vi "GameMode.vi"(8 "error in (no error)":errorcluster, 11 "UI in":refnum<class "UI.lvclass">) -> (0 "error out":errorcluster, 3 "UI out":refnum<class "UI.lvclass">)   [LabVIEW 2019]
uses:
  User Interface/UI.lvclass
  controls/DataIn.ctl
  controls/Tabuleiro.ctl
  controls/Table.ctl
  MatchDataClasses/MatchData/MatchData.lvclass
  User Interface/UI.lvclass/UI.ctl
  User Interface/setUIData.vi
  User Interface/getUIData.vi
  User Interface/setEmbeddedVI.vi
panel:
  in  "Player 2":string
  in  "Player 1":string
  in  "Difícil":bool
  in  "Fácil":bool
  in  "Médio":bool
  in  "Multiplayer Remoto":bool
  in  "Multiplayer Local":bool
  in  "Single Player":bool
  in  "Jogar":bool
  # "Modo de Jogo"
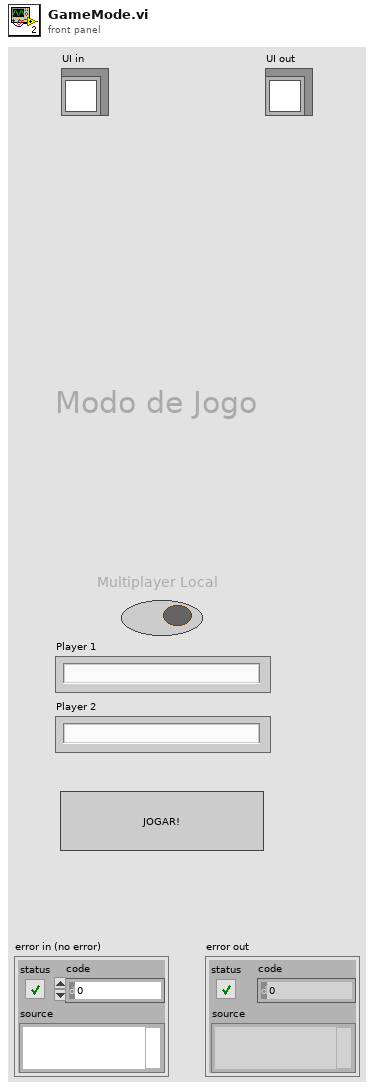
[diagram p1: front panel]
types:
  T1 = typedef "DataIn.ctl" = cluster{"Quem Joga":string, "Tabuleiro":T2, "GameOption":enum16{"Single Player", "Multiplayer local", "Multiplayer remoto", "Wait for Event", "Initialize", "Stop"}, "Turno":bool, "Player":string, "Player 1":string, "Player 2":string, "Dificuldade":enum16{"Easy", "Medium", "Hard"}, "Table":T3, "Row":u32, "Aceitar Convite":bool, "Inviter line":u32, "diretório":path, "Logout - panel close":bool, "StartGame":bool, "MatchData.lvclass":refnum<class "MatchData.lvclass">, "GameMode":enum16{"Single Easy", "Single Medium", "Single Hard", "Local", "Remote"}, "Level State":bool}
  T2 = typedef "Tabuleiro.ctl" = cluster{"(0,0)":string, "(1,0)":string, "(0,1)":string, "(1,1)":string, "(2,0)":string, "(1,2)":string, "(2,2)":string, "(0,2)":string, "(2,1) ":string}
  T3 = typedef "Table.ctl" = string[][]
  T4 = enum8{"Enabled", "Disabled", "Disabled and Grayed Out"}
  T5 = enum16{"Single Easy", "Single Medium", "Single Hard", "Local", "Remote"}
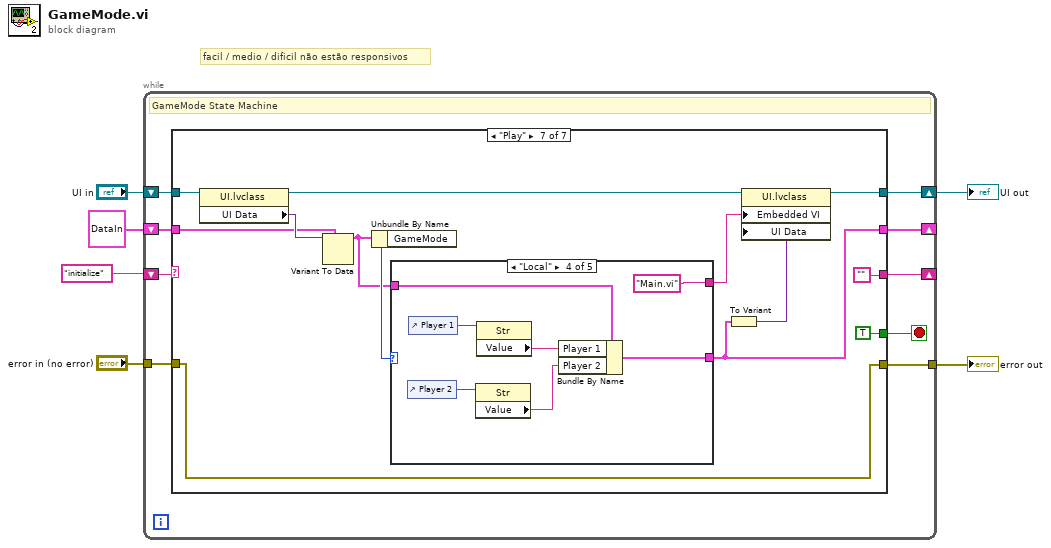
[diagram p0: block diagram]
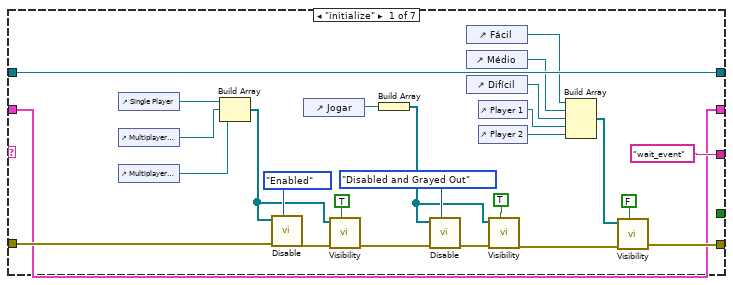
[diagram p2: hidden frame]
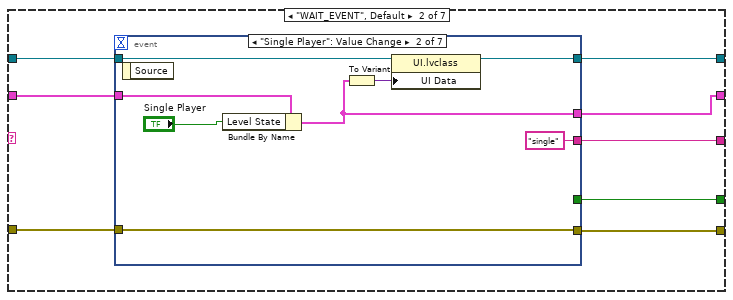
[diagram p3: hidden frame]
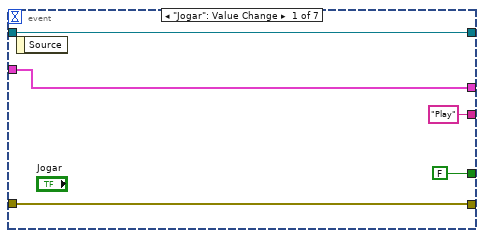
[diagram p4: hidden frame]
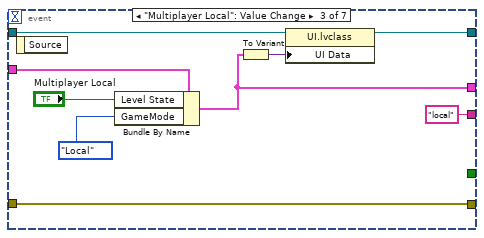
[diagram p5: hidden frame]
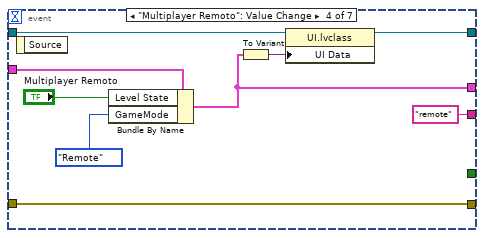
[diagram p6: hidden frame]
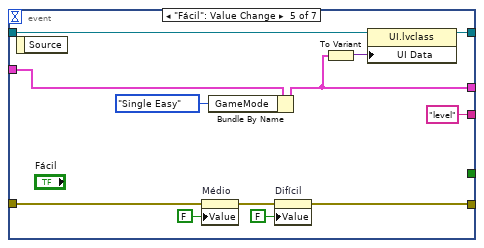
[diagram p7: hidden frame]
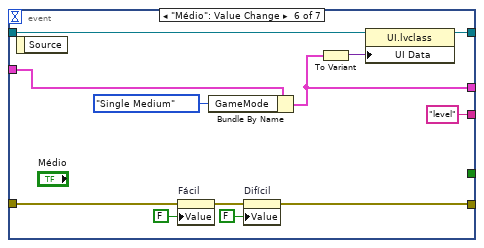
[diagram p8: hidden frame]
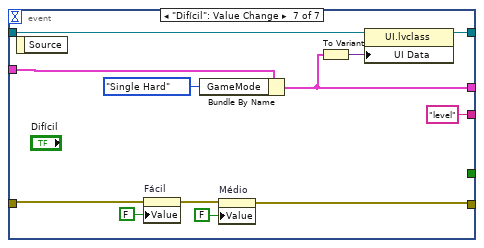
[diagram p9: hidden frame]
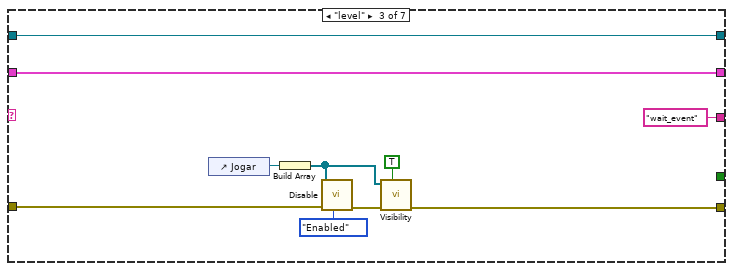
[diagram p10: hidden frame]
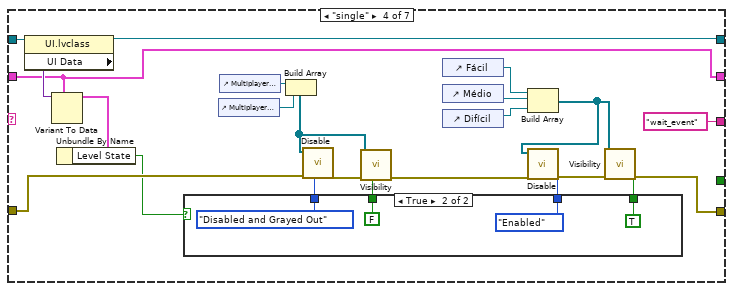
[diagram p11: hidden frame]
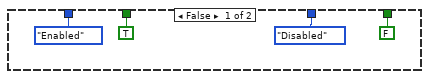
[diagram p12: hidden frame]
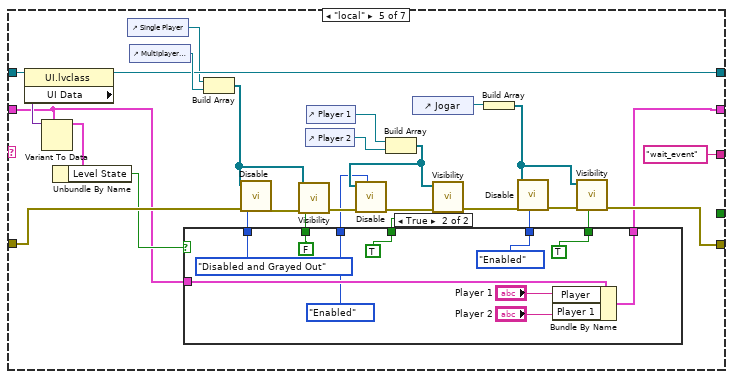
[diagram p13: hidden frame]
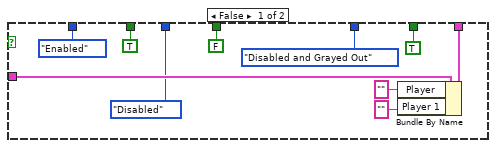
[diagram p14: hidden frame]
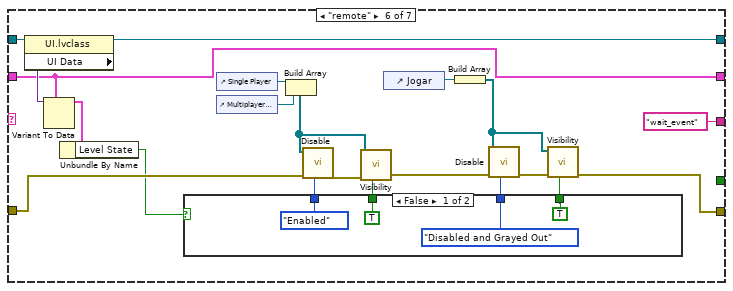
[diagram p15: hidden frame]
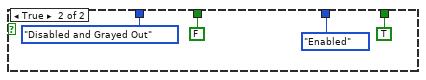
[diagram p16: hidden frame]
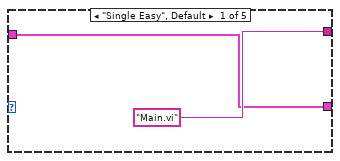
[diagram p17: hidden frame]
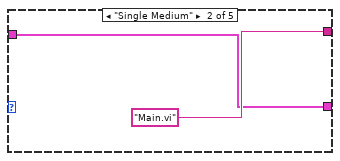
[diagram p18: hidden frame]
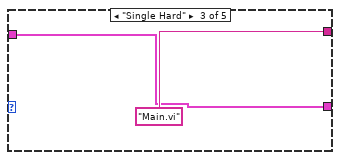
[diagram p19: hidden frame]
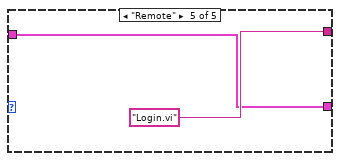
[diagram p20: hidden frame]
diagram:
  # "facil / medio / dificil não estão responsivos"
  n1 = while {
    shift-right: [w14] -> w5
    shift-left: "UI in" -> [w15]
    tunnel: [w13] -> w3
    tunnel: "error in (no error)" -> [w12]
    shift-right: [w11] -> _
    shift-left: "initialize" -> [w10]
    shift-right: [w7] -> _
    shift-left: T1 {"Quem Joga"="", "Tabuleiro"={"(0,0)"="", "(1,0)"="", "(0,1)"="", "(1,1)"="", "(2,0)"="", "(1,2)"="", "(2,2)"="", "(0,2)"="", "(2,1) "=""}, "GameOption"=enum."Multiplayer local", "Turno"=FALSE, "Player"="", "Player 1"="", "Player 2"="", "Dificuldade"=enum."Easy", "Table"=[], "Row"=0, "Aceitar Convite"=FALSE, "Inviter line"=0, "diretório"=path "", "Logout - panel close"=FALSE, "StartGame"=FALSE, "MatchData.lvclass"=refnum, "GameMode"=enum."Single Easy", "Level State"=FALSE} ("DataIn") -> [w8]
    stop <- w9 stop-if-true
    # "GameMode State Machine"
    n2 = case shown="\"Play\"" w10 {
      tunnel: w15 -> [w41 w49 w126 w133 w179 w221 w246]
      tunnel: [w41 w48 w126 w132 w178 w220 w248] -> w14
      tunnel: [w24 w47 w118 w134 w172 w213 w239] -> w13
      tunnel: w12 -> [w39 w46 w119 w142 w180 w222 w239]
      tunnel: ["wait_event" w45 "wait_event" "wait_event" "wait_event" "wait_event" ""] -> w11
      tunnel: [_ w44 _ _ _ _ TRUE] -> w9
      tunnel: w8 -> [w16 w43 w117 w130 w167 w209 w241]
      tunnel: [w16 w42 w117 w130 w166 w209 w237] -> w7
      frame "initialize" {
        n3 = control-ref of="Single Player"() -> (w37:refnum<vi>)
        n4 = control-ref of="Multiplayer Local"() -> (w36:refnum<vi>)
        n5 = control-ref of="Multiplayer Remoto"() -> (w35:refnum<vi>)
        n6 = Build Array(w37, w36, w35) -> (w33:refnum<vi>[])
        n7 = call "Disable.vi"("Disabled State"=T4."Enabled", "Error In"=w39, "Disable Controls"=w33) -> ("Error Out"=w34:errorcluster)  [unwired: 8 in]
        n8 = control-ref of="Jogar"() -> (w29:refnum<vi>)
        n9 = call "Visibility.vi"("Visible State"=TRUE, "Error In"=w34, "Visible Controls"=w33) -> ("Error Out"=w32:errorcluster)  [unwired: 8 in]
        n10 = Build Array(w29) -> (w27:refnum<vi>[])
        n11 = call "Disable.vi"("Disabled State"=T4."Disabled and Grayed Out", "Error In"=w32, "Disable Controls"=w27) -> ("Error Out"=w31:errorcluster)  [unwired: 8 in]
        n12 = control-ref of="Fácil"() -> (w18:refnum<vi>)
        n13 = control-ref of="Médio"() -> (w19:refnum<vi>)
        n14 = control-ref of="Difícil"() -> (w20:refnum<vi>)
        n15 = control-ref of="Player 1"() -> (w21:refnum<vi>)
        n16 = control-ref of="Player 2"() -> (w22:refnum<vi>)
        n17 = call "Visibility.vi"("Visible State"=TRUE, "Error In"=w31, "Visible Controls"=w27) -> ("Error Out"=w25:errorcluster)  [unwired: 8 in]
        n18 = Build Array(w18, w19, w20, w21, w22) -> (w17:refnum<vi>[])
        n19 = call "Visibility.vi"("Visible State"=FALSE, "Error In"=w25, "Visible Controls"=w17) -> ("Error Out"=w24:errorcluster)  [unwired: 8 in]
      }
      frame "WAIT_EVENT", Default {
        n20 = event shown="[1] \"Single Player\": Value Change" {
          selector: _ -> [_ _ _ _ _ _ _]
          dyn-events: _ -> [_ _ _ _ _ _ _]
          timeout: _ -> [_ _ _ _ _ _ _]
          tunnel: [w54 w59 w68 w77 w83 w96 w107] -> w48
          tunnel: w49 -> [w54 w60 w69 w78 w92 w95 w108]
          tunnel: [w53 w62 w71 w80 w88 w102 w114] -> w47
          tunnel: w46 -> [w53 w62 w71 w80 w89 w103 w116]
          tunnel: ["Play" "single" "local" "remote" "level" "level" "level"] -> w45
          tunnel: [FALSE _ _ _ _ _ _] -> w44
          tunnel: w43 -> [w50 w57 w66 w75 w85 w98 w111]
          tunnel: [w50 w55 w64 w73 w81 w93 w105] -> w42
          event "Jogar": Value Change {
            n21 = event-data() -> ()  [unwired: 1 in, 1 out]
          }
          event "Single Player": Value Change {
            n22 = event-data() -> ()  [unwired: 1 in, 1 out]
            n23 = Bundle By Name(cluster=w57, "Level State"="Single Player") -> (w55:T1)
            n24 = To Variant(anything=w55) -> (Variant=w58:variant)
            n25 = property class="UI.lvclass"(reference=w60, "UI Data"=w58) -> (reference out=w59:refnum<class "UI.lvclass">)  [unwired: 1 in, 1 out]
          }
          event "Multiplayer Local": Value Change {
            n26 = event-data() -> ()  [unwired: 1 in, 1 out]
            n27 = Bundle By Name(cluster=w66, "Level State"="Multiplayer Local", "GameMode"=T5."Local") -> (w64:T1)
            n28 = To Variant(anything=w64) -> (Variant=w67:variant)
            n29 = property class="UI.lvclass"(reference=w69, "UI Data"=w67) -> (reference out=w68:refnum<class "UI.lvclass">)  [unwired: 1 in, 1 out]
          }
          event "Multiplayer Remoto": Value Change {
            n30 = event-data() -> ()  [unwired: 1 in, 1 out]
            n31 = Bundle By Name(cluster=w75, "Level State"="Multiplayer Remoto", "GameMode"=T5."Remote") -> (w73:T1)
            n32 = To Variant(anything=w73) -> (Variant=w76:variant)
            n33 = property class="UI.lvclass"(reference=w78, "UI Data"=w76) -> (reference out=w77:refnum<class "UI.lvclass">)  [unwired: 1 in, 1 out]
          }
          event "Fácil": Value Change {
            n34 = event-data() -> ()  [unwired: 1 in, 1 out]
            n35 = property on="Médio" class="Bool (strict)"(error in=w89, "Value"=FALSE ("Médio")) -> (error out=w90:errorcluster)  [unwired: 1 in, 1 out]
            n36 = Bundle By Name(cluster=w85, "GameMode"=T5."Single Easy") -> (w81:T1)
            n37 = property on="Difícil" class="Bool (strict)"(error in=w90, "Value"=FALSE ("Difícil")) -> (error out=w88:errorcluster)  [unwired: 1 in, 1 out]
            n38 = To Variant(anything=w81) -> (Variant=w82:variant)
            n39 = property class="UI.lvclass"(reference=w92, "UI Data"=w82) -> (reference out=w83:refnum<class "UI.lvclass">)  [unwired: 1 in, 1 out]
          }
          event "Médio": Value Change {
            n40 = event-data() -> ()  [unwired: 1 in, 1 out]
            n41 = property on="Fácil" class="Bool (strict)"(error in=w103, "Value"=FALSE ("Fácil")) -> (error out=w104:errorcluster)  [unwired: 1 in, 1 out]
            n42 = Bundle By Name(cluster=w98, "GameMode"=T5."Single Medium") -> (w93:T1)
            n43 = property on="Difícil" class="Bool (strict)"(error in=w104, "Value"=FALSE ("Difícil")) -> (error out=w102:errorcluster)  [unwired: 1 in, 1 out]
            n44 = To Variant(anything=w93) -> (Variant=w94:variant)
            n45 = property class="UI.lvclass"(reference=w95, "UI Data"=w94) -> (reference out=w96:refnum<class "UI.lvclass">)  [unwired: 1 in, 1 out]
          }
          event "Difícil": Value Change {
            n46 = event-data() -> ()  [unwired: 1 in, 1 out]
            n47 = property on="Fácil" class="Bool (strict)"(error in=w116, "Value"=FALSE ("Fácil")) -> (error out=w115:errorcluster)  [unwired: 1 in, 1 out]
            n48 = Bundle By Name(cluster=w111, "GameMode"=T5."Single Hard") -> (w105:T1)
            n49 = property on="Médio" class="Bool (strict)"(error in=w115, "Value"=FALSE ("Médio")) -> (error out=w114:errorcluster)  [unwired: 1 in, 1 out]
            n50 = To Variant(anything=w105) -> (Variant=w106:variant)
            n51 = property class="UI.lvclass"(reference=w108, "UI Data"=w106) -> (reference out=w107:refnum<class "UI.lvclass">)  [unwired: 1 in, 1 out]
          }
        }
      }
      frame "level" {
        n52 = control-ref of="Jogar"() -> (w123:refnum<vi>)
        n53 = Build Array(w123) -> (w122:refnum<vi>[])
        n54 = call "Disable.vi"("Disabled State"=T4."Enabled", "Error In"=w119, "Disable Controls"=w122) -> ("Error Out"=w124:errorcluster)  [unwired: 8 in]
        n55 = call "Visibility.vi"("Visible State"=TRUE, "Error In"=w124, "Visible Controls"=w122) -> ("Error Out"=w118:errorcluster)  [unwired: 8 in]
      }
      frame "single" {
        n56 = property class="UI.lvclass"(reference=w133) -> (reference out=w132:refnum<class "UI.lvclass">, "UI Data"=w131:variant)  [unwired: 1 in, 1 out]
        n57 = Variant To Data(type=w130, Variant=w131) -> (data=w129:T1)  [unwired: 1 in, 1 out]
        n58 = Unbundle By Name(w129) -> ("Level State"=w128:bool)
        n59 = case shown="True" w128 {
          tunnel: [T4."Enabled" ("Disabled State") T4."Disabled and Grayed Out" ("Disabled State")] -> w148
          tunnel: [TRUE ("Visible State") FALSE ("Visible State")] -> w143
          tunnel: [FALSE ("Visible State") TRUE ("Visible State")] -> w141
          tunnel: [T4."Disabled" ("Disabled State") T4."Enabled" ("Disabled State")] -> w135
          frame False {
          }
          frame True {
          }
        }
        n60 = control-ref of="Multiplayer Remoto"() -> (w146:refnum<vi>)
        n61 = control-ref of="Multiplayer Local"() -> (w147:refnum<vi>)
        n62 = Build Array(w147, w146) -> (w144:refnum<vi>[])
        n63 = call "Disable.vi"("Disabled State"=w148, "Error In"=w142, "Disable Controls"=w144) -> ("Error Out"=w145:errorcluster)  [unwired: 8 in]
        n64 = call "Visibility.vi"("Visible State"=w143, "Error In"=w145, "Visible Controls"=w144) -> ("Error Out"=w137:errorcluster)  [unwired: 8 in]
        n65 = control-ref of="Fácil"() -> (w140:refnum<vi>)
        n66 = control-ref of="Médio"() -> (w139:refnum<vi>)
        n67 = control-ref of="Difícil"() -> (w138:refnum<vi>)
        n68 = Build Array(w140, w139, w138) -> (w127:refnum<vi>[])
        n69 = call "Disable.vi"("Disabled State"=w135, "Error In"=w137, "Disable Controls"=w127) -> ("Error Out"=w136:errorcluster)  [unwired: 8 in]
        n70 = call "Visibility.vi"("Visible State"=w141, "Error In"=w136, "Visible Controls"=w127) -> ("Error Out"=w134:errorcluster)  [unwired: 8 in]
      }
      frame "local" {
        n71 = property class="UI.lvclass"(reference=w179) -> (reference out=w178:refnum<class "UI.lvclass">, "UI Data"=w177:variant)  [unwired: 1 in, 1 out]
        n72 = Variant To Data(type=w167, Variant=w177) -> (data=w169:T1)  [unwired: 1 in, 1 out]
        n73 = Unbundle By Name(w169) -> ("Level State"=w168:bool)
        n74 = control-ref of="Single Player"() -> (w176:refnum<vi>)
        n75 = control-ref of="Multiplayer Remoto"() -> (w184:refnum<vi>)
        n76 = case shown="True" w168 {
          tunnel: [T4."Enabled" ("Disabled State") T4."Disabled and Grayed Out" ("Disabled State")] -> w185
          tunnel: [TRUE ("Visible State") FALSE ("Visible State")] -> w181
          tunnel: [TRUE ("Visible State") TRUE ("Visible State")] -> w171
          tunnel: [T4."Disabled and Grayed Out" ("Disabled State") T4."Enabled" ("Disabled State")] -> w170
          tunnel: w167 -> [w192 w202]
          tunnel: [w189 w199] -> w166
          tunnel: [FALSE ("Visible State") TRUE ("Visible State")] -> w162
          tunnel: [T4."Disabled" ("Disabled State") T4."Enabled" ("Disabled State")] -> w158
          frame False {
            n77 = Bundle By Name(cluster=w192, "Player"="", "Player 1"="") -> (w189:T1)
          }
          frame True {
            n78 = Bundle By Name(cluster=w202, "Player"="Player 1", "Player 1"="Player 2") -> (w199:T1)
          }
        }
        n79 = Build Array(w176, w184) -> (w182:refnum<vi>[])
        n80 = call "Disable.vi"("Disabled State"=w185, "Error In"=w180, "Disable Controls"=w182) -> ("Error Out"=w183:errorcluster)  [unwired: 8 in]
        n81 = call "Visibility.vi"("Visible State"=w181, "Error In"=w183, "Visible Controls"=w182) -> ("Error Out"=w161:errorcluster)  [unwired: 8 in]
        n82 = control-ref of="Player 2"() -> (w165:refnum<vi>)
        n83 = control-ref of="Player 1"() -> (w164:refnum<vi>)
        n84 = Build Array(w164, w165) -> (w159:refnum<vi>[])
        n85 = call "Disable.vi"("Disabled State"=w158, "Error In"=w161, "Disable Controls"=w159) -> ("Error Out"=w160:errorcluster)  [unwired: 8 in]
        n86 = control-ref of="Jogar"() -> (w174:refnum<vi>)
        n87 = call "Visibility.vi"("Visible State"=w162, "Error In"=w160, "Visible Controls"=w159) -> ("Error Out"=w163:errorcluster)  [unwired: 8 in]
        n88 = Build Array(w174) -> (w173:refnum<vi>[])
        n89 = call "Disable.vi"("Disabled State"=w170, "Error In"=w163, "Disable Controls"=w173) -> ("Error Out"=w175:errorcluster)  [unwired: 8 in]
        n90 = call "Visibility.vi"("Visible State"=w171, "Error In"=w175, "Visible Controls"=w173) -> ("Error Out"=w172:errorcluster)  [unwired: 8 in]
      }
      frame "remote" {
        n91 = property class="UI.lvclass"(reference=w221) -> (reference out=w220:refnum<class "UI.lvclass">, "UI Data"=w219:variant)  [unwired: 1 in, 1 out]
        n92 = Variant To Data(type=w209, Variant=w219) -> (data=w208:T1)  [unwired: 1 in, 1 out]
        n93 = Unbundle By Name(w208) -> ("Level State"=w207:bool)
        n94 = case shown="False" w207 {
          tunnel: [T4."Enabled" ("Disabled State") T4."Disabled and Grayed Out" ("Disabled State")] -> w226
          tunnel: [TRUE ("Visible State") FALSE ("Visible State")] -> w223
          tunnel: [TRUE ("Visible State") TRUE ("Visible State")] -> w212
          tunnel: [T4."Disabled and Grayed Out" ("Disabled State") T4."Enabled" ("Disabled State")] -> w211
          frame False {
          }
          frame True {
          }
        }
        n95 = control-ref of="Single Player"() -> (w218:refnum<vi>)
        n96 = control-ref of="Multiplayer Local"() -> (w210:refnum<vi>)
        n97 = Build Array(w218, w210) -> (w224:refnum<vi>[])
        n98 = call "Disable.vi"("Disabled State"=w226, "Error In"=w222, "Disable Controls"=w224) -> ("Error Out"=w225:errorcluster)  [unwired: 8 in]
        n99 = call "Visibility.vi"("Visible State"=w223, "Error In"=w225, "Visible Controls"=w224) -> ("Error Out"=w214:errorcluster)  [unwired: 8 in]
        n100 = control-ref of="Jogar"() -> (w216:refnum<vi>)
        n101 = Build Array(w216) -> (w215:refnum<vi>[])
        n102 = call "Disable.vi"("Disabled State"=w211, "Error In"=w214, "Disable Controls"=w215) -> ("Error Out"=w217:errorcluster)  [unwired: 8 in]
        n103 = call "Visibility.vi"("Visible State"=w212, "Error In"=w217, "Visible Controls"=w215) -> ("Error Out"=w213:errorcluster)  [unwired: 8 in]
      }
      frame "Play" {
        n104 = property class="UI.lvclass"(reference=w246) -> (reference out=w245:refnum<class "UI.lvclass">, "UI Data"=w244:variant)  [unwired: 1 in, 1 out]
        n105 = Variant To Data(type=w241, Variant=w244) -> (data=w238:T1)  [unwired: 1 in, 1 out]
        n106 = Unbundle By Name(w238) -> ("GameMode"=w243:T5)
        n107 = case shown="\"Local\"" w243 {
          tunnel: ["Main.vi" ("String <Replace Me>") "Main.vi" ("String <Replace Me>") "Main.vi" ("String <Replace Me>") "Main.vi" ("String <Replace Me>") "Login.vi" ("String <Replace Me>")] -> w242
          tunnel: w238 -> [w249 w251 w253 w258 w262]
          tunnel: [w249 w251 w253 w255 w262] -> w237
          frame "Single Easy", Default {
          }
          frame "Single Medium" {
          }
          frame "Single Hard" {
          }
          frame "Local" {
            n108 = control-ref of="Player 2"() -> (w259:refnum<vi>)
            n109 = control-ref of="Player 1"() -> (w260:refnum<vi>)
            n110 = property class="Str"(reference=w259) -> ("Value"=w256:string)  [unwired: 1 in, 2 out]
            n111 = property class="Str"(reference=w260) -> ("Value"=w257:string)  [unwired: 1 in, 2 out]
            n112 = Bundle By Name(cluster=w258, "Player 1"=w257, "Player 2"=w256) -> (w255:T1)
          }
          frame "Remote" {
          }
        }
        n113 = To Variant(anything=w237) -> (Variant=w236:variant)
        n114 = property class="UI.lvclass"(reference=w245, "Embedded VI"=w242, "UI Data"=w236) -> (reference out=w248:refnum<class "UI.lvclass">)  [unwired: 1 in, 1 out]
      }
    }
  }
  "UI out" <- w5
  "error out" <- w3
